vi "Convert_Hex_to_Normal_String_2010.vi"(9 "Initial Hex String":string="Hello World!") -> (3 "Normal String - Format into String Method":string)   [LabVIEW 2017]
panel:
  out "Normal String - Number to Hexadecimal String Method":string
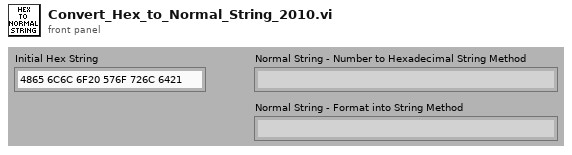
[diagram p1: front panel]
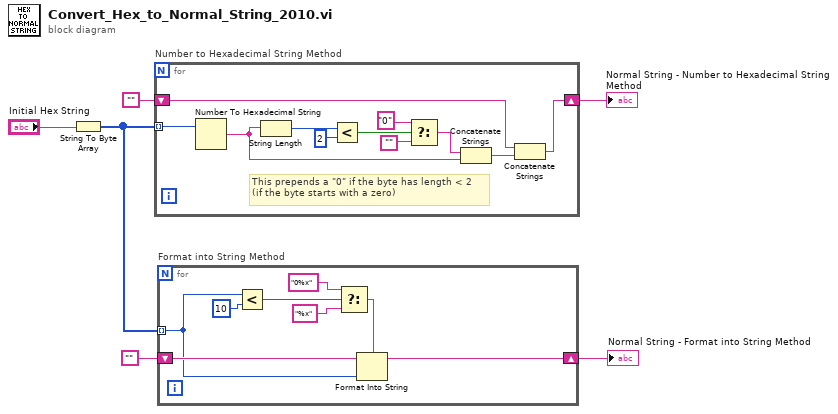
[diagram p0: block diagram]
diagram:
  n1 = String To Byte Array(string="Initial Hex String") -> (unsigned byte array=w3:u8[])
  n2 = for "Number to Hexadecimal String Method" {
    shift-right: [w17] -> w5
    shift-left: "" -> [w7]
    tunnel: w3 -> [w8] mode=indexing
    # "This prepends a \"0\" if the byte has length < 2\n(if the byte starts with a zero)"
    n3 = Number To Hexadecimal String(2:w8) -> (0:w10:string)  [unwired: 1 in]
    n4 = String Length(string=w10) -> (length=w16:i32)
    n5 = Less?(x=w16, y=2) -> (x < y?=w14:bool)
    n6 = Select(t="0", s=w14, f="") -> (s? t:f=w11:string)
    n7 = Concatenate Strings(w11, w10) -> (w9:string)
    n8 = Concatenate Strings(w7, w9) -> (w17:string)
  }
  "Normal String - Number to Hexadecimal String Method" <- w5
  n9 = for "Format into String Method" {
    tunnel: w3 -> [w19] mode=indexing
    shift-right: [w18] -> w1
    shift-left: "" -> [w20]
    n10 = Less?(x=w19, y=u8 10) -> (x < y?=w24:bool)
    n11 = Select(t="0%x" ("format string"), s=w24, f="%x" ("format string")) -> (s? t:f=w21:string)
    n12 = Format Into String(format string=w21, initial string=w20, w19) -> (resulting string=w18:string)  [unwired: 1 in, 1 out]
  }
  "Normal String - Format into String Method" <- w1
